vi "LSMcontroller_v57.vi"() -> ()   [LabVIEW 2015] (continued)
  out "graph1":dbl[](graph)=[-0.0018560309667373077, -0.0018495913478545844, -0.0010736164951231331, -0.001495411962387152, -0.0016886007197899743, -0.0017819752829382196, -0.002049219731125049, -0.0016853808861924334, -0.0013730590644991025, -0.0016853808995801955, -0.0015823469014139846, -0.0019494055502582341, -0.0022907056851545348, -0.0020041423733346162, -0.002042780100600794, -0.001814173402963206, -0.001997702724765986, -0.002136154668405652, -0.002451696299831383, -0.0024710151832550765, -0.0021297150413738565, -0.002165132985683158, -0.0019429659144952892, -0.0021908914903178813, -0.0024291576351970433, -0.002606247318908572, -0.0019204272195929661, -0.0018946687219431623, -0.002097516918438487, -0.0021844518574653192, -0.002290705653722398, -0.0020299008616711943, -0.001859250800916925, -0.0015630280249752104, -0.001852811174467206, -0.0017884149093879388, -0.001955845166812651, -0.0018302724667591975, -0.0012957835738779976, -0.0013923779356991872, -0.0015018515911651776, -0.0015404893353115768, -0.0016467431501951068, -0.0016789412929210813, -0.0015533685742411762, -0.0014116968284361064, -0.00147931290557608, -0.001682161101489328, -0.002023461216595024, -0.0021941113128559663, -0.0019429659086745233, -0.0014567741996143013, -0.0017916347202844918, -0.0021393744961824266, -0.0021941113081993535, -0.0022327490517636763, -0.0023132443812210112, -0.002129715041955933, -0.002149033914320171, -0.002216649982728995, -0.0024645755731035023, -0.002760798340314068, -0.0022295292594935747, -0.00198482348525431, -0.0021168357878923417, -0.002065318789682351, -0.0024259378161514177, -0.002239188695093617, -0.0022134301700862126, -0.001917207420920022, -0.0015469289664179087, -0.0017626564193051308, -0.0020459999179001896, -0.0021136160084279255, -0.0018689102173084394, -0.0013408609433099628, -0.0014406751602655276, -0.001495411946089007, -0.0016982601588824765, -0.001820613036979921, -0.0014213562669465319, -0.001437455345876515, -0.0012088486348511651, -0.0014503345714183525, -0.0016467431612545624, -0.0018012941704364494, -0.0016918205167166889, -0.0016596224083332345, -0.0016370837058639154, -0.0016950403252849356, -0.002084637672523968, -0.002326123615493998, -0.0023068047373089938, -0.0022585075575625524, -0.00199126310297288, -0.002107176355784759, -0.002165133003727533, -0.0026384454587241634, -0.0025676095741800965, -0.0025225321960169822, -0.0021264952316414564, -0.0020427801075857135, -0.0021200556465191768, -0.002245628290693276, -0.002390519853797741, -0.0022746066143736242, -0.0020910772954812274, -0.0017851950967451558, -0.0017465573363006114, -0.0018817894713720306, -0.0021619131858460604, -0.0017916347179561852, -0.001736897912924178, -0.0016048855806002392, -0.0013344213337404653, -0.0013794987014262006, -0.001804513976094313, -0.0018334922881331295, -0.0016821610782062635, -0.0012861241400241852, -0.0011605514463735745, -0.0016467431490309536, -0.0018334922892972827, -0.0017948545346735045, -0.0018528111593332142, -0.0015662478364538402, -0.0017948545276885851, -0.0018495913362130522, -0.00211683580360841, -0.0022907056659460068, -0.002065318794338964, -0.002100736728752963, -0.001965504598338157, -0.001923647031071596, -0.002380860450793989, -0.0025160925590898844, -0.0024516962975030766, -0.0021973311249166728, -0.0021425942954374478, -0.0021039565571118147, -0.002480674621765502, -0.0024581359419971706, -0.002406618939130567, -0.0020653187792049723, -0.0020331206818809734, -0.0019011083693476394, -0.0024066189402947202, -0.002100736736319959, -0.001959064974216744, -0.0016757214703829958, -0.0015243902738438918, -0.001749777131481096, -0.001827052648877725, -0.0015662478102603926, -0.0017046997835859657, -0.0015501487703295424, -0.0013891581393545493, -0.0013762788905296475, -0.0014213562599616125, -0.00181739320687484, -0.001666062013246119, -0.0017240186640992761, -0.0012829043267993257, -0.0016274242772487924, -0.0016821611020714044, -0.0021329348516883327, -0.0020009225263493136, -0.002216649993788451, -0.0018399319046875462, -0.0016950403217924758, -0.002116835783235729, -0.0023357830644818024, -0.002493553873500787, -0.002644885074696504, -0.0022230896214023234, -0.0021039565443061294, -0.00202668106299825, -0.002371201001224108, -0.002718940763734281, -0.0023583217366831377, -0.002239188690437004, -0.001988043275196105, -0.001933306478895247, -0.0023969594959635286, -0.002149033925961703, -0.0019333064742386341, -0.0017851950996555389, -0.0015662478434387594, -0.001572687451262027, -0.0017207988345762715, -0.001968724424368702, -0.001749777148361318, -0.0017111394059611484, -0.0011991891922662034, -0.0012957835855195298, -0.0015694676392013207, -0.0018431517033604904, -0.00160810538160149, -0.001669281840440817, -0.0014857525273691862, -0.001495411968207918, -0.0017143592133652419, -0.0020266810234170407, -0.0022295292478520423, -0.0019751640438335017, -0.0016821610962506383, -0.00206209899391979, -0.0020910772978095338, -0.0025579501484753564, -0.0023454424826195464, -0.0021651330019813032, -0.0020942971110343932, -0.0021264952316414564, -0.002206990561098792, -0.0025386312487535177, -0.0024323774583172053, -0.002242408492020331, -0.0021361546911066397, -0.0019429659011075274, -0.0021071763639338315, -0.0024806746386457235, -0.0022552877361886204, -0.0019333064934471621, -0.0015565884031821043, -0.0018656904040835797, -0.0017368979088496416, -0.0020620989764574913, -0.002004142368095927, -0.0018141734122764318, -0.0014471147704171016, -0.0011025947914458812, -0.0015501487709116192, -0.0018624705949332565, -0.0017948545253602787, -0.00177231585199479, -0.0013537401973735541, -0.0013698392553487793, -0.0016628422040957957, -0.0017401177121791989, -0.00198482348350808, -0.0020395603036740795, -0.0018399319052696229, -0.0015018515754491092, -0.0017916347266873345, -0.0021812320401659235, -0.00237764063233044, -0.002216649978654459, -0.002123275414924137, -0.001949405528139323, -0.0019977027032291516, -0.002387300063855946, -0.0025515104917576536, -0.002274606619030237, -0.002081417862791568, -0.002078198051312938, -0.001981603662716225, -0.002487114255782217, -0.002786556836217642, -0.0020588791550835593, -0.0017690960131585597, -0.001769096020143479, -0.0019300866511184722, -0.0021329348592553287, -0.0022681669978192077, -0.0018946687231073155, -0.0015147308318410068, -0.0013601798203308135, -0.0015630280249752104, -0.002039560312987305, -0.0021973311225883664, -0.00174977716000285, -0.0012957835773704574, -0.0012378269532928243, -0.0014342355192638935, -0.0020653187891002743, -0.0018399319058516994, -0.0015372695308178664, -0.001476093094679527, -0.00159200633817818, -0.0017690960387699306, -0.0017562167765572667, -0.0020331206731498243, -0.002190891476930119, -0.001936526307836175, -0.0016467431496130303, -0.0016338639007881283, -0.0022102103638462723, -0.0023776406107936052, -0.0023905198776628823, -0.002152253762469627, -0.001859250787529163, -0.002155473546590656, -0.00242593782953918, -0.0023357830609893426, -0.002393739692051895, -0.0021522537450073286, -0.00203634048870299, -0.0020041423657676206, -0.0021232754172524435, -0.0023390028806170447, -0.0022746066277613865, -0.001868910220800899, -0.0016692818503361195, -0.0017207988328300416, -0.001881789463222958, -0.0019429659412708133, -0.0020266810309840367, -0.0017272384563693777, -0.001334421323845163, -0.0012700250651687384, -0.001740117723820731, -0.0018656904302770273, -0.001794854526524432, -0.001469653451931663, -0.0015437091555213557, -0.0015791270794579758, -0.0017272384988609702, -0.0017529969615861774, -0.002013801789144054, -0.0020266810426255687, -0.0016821610735496507, -0.0016692818270530553, -0.0017723158199805767, -0.0023100245353998615, -0.002416278381133452, -0.002290705683408305, -0.0018689102382631973, -0.0017594366031698882, -0.0021876716788392513, -0.002458135940833017, -0.002361541569116525, -0.0023293434327933938, -0.0019526253320509568, -0.0018431517231510951, -0.0021168357849819584, -0.0024903340463060886, -0.00241305856325198, -0.002332563240779564, -0.001785195113043301, -0.001843151740031317, -0.0017980743205407634, -0.0019590649631572887, -0.00209751692134887, -0.0019880433013895527, -0.0015565884084207937, -0.0013633996300632134, -0.0015501487522851676, -0.0017143592156935482, -0.00209107730537653, -0.0016789412766229361, -0.0013666194613324478, -0.0013633996393764391, -0.0012668052542721853, -0.001556588388630189, -0.0019075479550519957, -0.0018238328368170187, -0.001756216786452569, -0.0014986317686270921, -0.0014277958963066339, -0.0017916347336722539, -0.0019397461105836555, -0.002210210368502885, -0.002132934860419482, -0.0018817894748644904, -0.0018656904192175716, -0.0019880432955687866, -0.002033120676060207, -0.0023551019409205763, -0.002467795368283987, -0.002052439529215917, -0.0018173932161880658, -0.0022166499897139148, -0.0023840802599443124, -0.0024581359291914852, -0.0024549161351751538, -0.0023712010233430192, -0.0020009225455578416, -0.0018334922770736738, -0.001942965938942507, -0.001939746110001579, -0.002329343447345309, -0.0020073621690971776, -0.0017916347255231813, -0.0015082911960780621, -0.00143423551809974, -0.0017240186623530462, -0.0019751640473259615, -0.0019107677799183875, -0.001572687461739406, -0.0012925637559965252, -0.0010736165021080523, -0.0015726874460233375, -0.0018270526523701846, -0.0018689102242933587, -0.001685380867565982, -0.0015501487615983934, -0.001347300586057827, -0.0016370837099384517, -0.0019977027317509056, -0.002097516935900785, -0.0020717584155499937, -0.0016757214447716252, -0.0018206130363978446, -0.0020814178476575764, -0.002345442486112006, -0.0026642039592843503, -0.002264947179937735, -0.0019043281738413498, -0.002161913178279065, -0.002149033920140937, -0.0024194981885375453, -0.0025579501315951348, -0.002306804757681675, -0.002007362169679254, -0.001933306460850872, -0.0021844518580473957, -0.002184451878420077, -0.002271386809879914, -0.00211039618588984, -0.00177231585199479, -0.0015759072575019673, -0.0017143592203501612, -0.0017111393983941525, -0.0019590649823658167, -0.001791634718538262, -0.0016435233206721022, -0.0011637712555238977, -0.001453554396284744, -0.0017336780938785523, -0.0016982601548079402, -0.0018656904180534184, -0.001563028022646904, -0.0011573316162684932, -0.0015726874658139422, -0.0014567742095096038, -0.0018721300427569077, -0.002107176362769678, -0.0019461857079295442, -0.0019397461030166597, -0.0018045139574678615, -0.0019204272172646598, -0.0019912631140323357, -0.002187671684077941, -0.0024291576375253497, -0.0023035849432926623, -0.0020653187989955767, -0.0020717584114754574, -0.002123275409685448, -0.0023390028876019643, -0.002622346395510249, -0.0023261236131656917, -0.002252067932859063, -0.001865690387203358, -0.0020041423477232456, -0.0021329348761355504, -0.0022778264153748753, -0.0021103961765766145, -0.001959064967231825, -0.001717579016694799, -0.0014986317593138664, -0.001627424283651635, -0.0018914489058079198, -0.0018367120838956906, -0.0014406751457136124, -0.0015501487586880103, -0.0013022232073126362, -0.001421356256469153, -0.0016982601478230208, -0.0015501487703295424, -0.0018045139615423978, -0.001582346884533763, -0.0013440807693405076, -0.0015179506508866325, -0.0018302724696695805, -0.002000922540901229, -0.0018431517150020228, -0.001823832843801938, -0.0017980743595398963, -0.0018817894667154179, -0.0019268668530276045, -0.0022424084757221865, -0.0026481048861751334, -0.002406618953682482, -0.002087857477017678, -0.0018431517371209339, -0.0024066189589211718, -0.0023647613829234615, -0.002284266062779352, -0.002499993511009961, -0.0021908914734376592, -0.001904328142409213, -0.0021071763546206056, -0.0021490339195588603, -0.002522532190196216, -0.002113615990965627, -0.0016499629808822648, -0.0016338638897286728, -0.0017368979076854885, -0.00202346122416202, -0.001852811149437912]
  in  "graph1list":u16(ring) items=["PMT"]
  out "Cmembrane":dbl
  in  "fitpoints":dbl=10.0
  out "Racces (MOhm)":dbl
  out "Rmembrane (MOhm)":dbl
  in  "set as Rp?":bool
  out "Ifit":dbl[](graph)
  in  "readpatch":bool
  in  "Voltage Clamp":bool=TRUE
  in  "OCgain":sgl(ring)=5.0 caption="Output Current gain (mV/pA)" items=["2K"=2000, "1K"=1000, "500"=500, "200"=200, "100"=100, "50"=50, "20"=20, "10"=10, "5"=5, "2"=2, "1"=1, "0.5"=0.5, "0.2"=0.2, "0.1"=0.1, "0.05"=0.05, "0.02"=0.02, "0.01"=0.01, "0.005"=0.005]
  in  "holdon":bool
  out "CC_ICgain":dbl(ring)=10.0 caption="Current Clamp \ninput current gain (pA/mV)" items=["0.1"=10.0, "10"=0.1]
  out "Patch readout":dbl[][](graph)=[[-19.129690948880636, -18.936502231865173, -19.129690948880636, -19.065294709927485, -19.065294709927485, -19.097492829410562, -19.065294709927485, -19.000898470922337, -19.065294709927485, -19.065294709927485, -19.097492829410562, -19.129690948880636, -19.065294709927485, -19.22628530721287, -19.065294709927485, -19.033096590431416, -19.000898470922337, -19.129690948880636, -19.065294709927485, -19.000898470922337, -19.097492829410562, -19.097492829410562, -19.129690948880636, -19.097492829410562, -19.065294709927485, -19.19408718778179, -18.96870035140026, -19.033096590431416, -19.097492829410562, -19.033096590431416, -19.065294709927485, -19.065294709927485, -19.129690948880636, -19.097492829410562, -19.129690948880636, -19.16188906833771, -19.065294709927485, -19.065294709927485, -19.16188906833771, -19.16188906833771, -19.065294709927485, -19.129690948880636, -19.097492829410562, -19.033096590431416, -19.065294709927485, -19.129690948880636, -19.065294709927485, -19.033096590431416, -19.033096590431416, -19.129690948880636, -19.19408718778179, -19.065294709927485, -9.148273285922594, -9.212669532972436, -9.180471409454158, -9.083877038819596, -9.148273285922594, -9.148273285922594, -9.083877038819596, -9.148273285922594, -9.180471409454158, -9.180471409454158, -9.180471409454158, -9.212669532972436, -9.212669532972436, -9.180471409454158, -9.212669532972436, -9.11607516237774, -9.244867656477426, -9.11607516237774, -9.212669532972436, -9.244867656477426, -9.244867656477426, -9.11607516237774, -9.148273285922594, -9.212669532972436, -9.148273285922594, -9.212669532972436, -9.212669532972436, -9.180471409454158, -9.180471409454158, -9.277065779969131, -9.309263903447553, -9.244867656477426, -9.180471409454158, -9.180471409454158, -9.148273285922594, -9.244867656477426, -9.212669532972436, -9.244867656477426, -9.083877038819596, -9.212669532972436, -9.277065779969131, -9.244867656477426, -9.180471409454158, -9.11607516237774, -9.180471409454158, -9.212669532972436, -9.212669532972436, -9.212669532972436, -9.11607516237774, -9.180471409454158, -19.065294709927485, -19.097492829410562, -19.097492829410562, -19.16188906833771, -19.16188906833771, -19.033096590431416, -19.065294709927485, -19.129690948880636, -19.129690948880636, -19.097492829410562, -19.033096590431416, -19.258483426630953, -19.129690948880636, -19.033096590431416, -19.097492829410562, -19.129690948880636, -19.097492829410562, -19.19408718778179, -19.16188906833771, -19.097492829410562, -19.033096590431416, -19.000898470922337, -19.065294709927485, -19.16188906833771, -19.129690948880636, -19.129690948880636, -19.065294709927485, -19.033096590431416, -19.097492829410562, -19.097492829410562, -19.097492829410562, -18.96870035140026, -19.097492829410562, -19.19408718778179, -19.097492829410562, -19.065294709927485, -19.097492829410562, -19.129690948880636, -19.16188906833771, -19.033096590431416, -19.065294709927485, -19.129690948880636, -19.129690948880636, -19.065294709927485, -19.065294709927485, -19.033096590431416, -19.16188906833771, -19.097492829410562, -19.19408718778179, -19.000898470922337, -9.148273285922594, -9.148273285922594, -9.148273285922594, -9.019480791663437, -9.180471409454158, -9.277065779969131, -9.148273285922594, -9.148273285922594, -9.180471409454158, -9.180471409454158, -9.11607516237774, -9.180471409454158, -9.180471409454158, -9.11607516237774, -9.083877038819596, -9.341462026912685, -9.180471409454158, -9.11607516237774, -9.11607516237774, -9.212669532972436, -9.11607516237774, -9.11607516237774, -9.083877038819596, -9.11607516237774, -9.180471409454158, -9.11607516237774, -9.11607516237774, -9.244867656477426, -9.180471409454158, -9.180471409454158, -9.244867656477426, -9.180471409454158, -9.180471409454158, -9.180471409454158, -9.180471409454158, -9.180471409454158, -9.148273285922594, -9.11607516237774, -9.180471409454158, -9.212669532972436, -9.180471409454158, -9.148273285922594, -9.083877038819596, -9.11607516237774, -9.180471409454158, -9.148273285922594, -9.148273285922594, -9.148273285922594, -9.212669532972436, -9.11607516237774, -19.000898470922337, -19.065294709927485, -19.097492829410562, -19.129690948880636, -19.097492829410562, -18.936502231865173, -18.96870035140026, -19.097492829410562, -19.065294709927485, -19.097492829410562, -19.22628530721287, -19.065294709927485, -19.000898470922337, -19.000898470922337, -19.16188906833771, -19.065294709927485, -18.96870035140026, -19.097492829410562, -19.129690948880636, -19.065294709927485, -19.097492829410562, -19.129690948880636, -19.129690948880636, -19.16188906833771, -19.129690948880636, -19.129690948880636, -19.065294709927485, -19.000898470922337, -19.065294709927485, -19.065294709927485, -19.129690948880636, -19.033096590431416, -19.129690948880636, -19.065294709927485, -19.129690948880636, -19.097492829410562, -18.96870035140026, -19.097492829410562, -19.097492829410562, -19.065294709927485, -19.097492829410562, -19.129690948880636, -19.000898470922337, -19.033096590431416, -19.097492829410562, -19.097492829410562, -19.033096590431416, -18.96870035140026, -19.000898470922337, -19.129690948880636, -9.019480791663437, -9.083877038819596, -9.11607516237774, -9.083877038819596, -9.148273285922594, -9.309263903447553, -9.148273285922594, -9.11607516237774, -9.180471409454158, -9.180471409454158, -9.148273285922594, -9.148273285922594, -9.212669532972436, -9.019480791663437, -9.180471409454158, -9.148273285922594, -9.212669532972436, -9.051678915248162, -9.180471409454158, -9.212669532972436, -9.148273285922594, -9.212669532972436, -9.148273285922594, -9.11607516237774, -9.180471409454158, -9.212669532972436, -9.11607516237774, -9.083877038819596, -9.180471409454158, -9.11607516237774, -9.148273285922594, -9.083877038819596, -9.244867656477426, -9.212669532972436, -9.11607516237774, -9.11607516237774, -9.11607516237774, -9.148273285922594, -9.11607516237774, -9.11607516237774, -9.148273285922594, -9.180471409454158, -9.180471409454158, -9.051678915248162, -9.083877038819596, -9.083877038819596, -9.244867656477426, -9.083877038819596, -9.051678915248162, -9.148273285922594, -19.065294709927485, -19.065294709927485, -19.000898470922337, -19.000898470922337, -19.097492829410562, -19.065294709927485, -19.000898470922337, -19.097492829410562, -19.097492829410562, -19.033096590431416, -19.033096590431416, -19.033096590431416, -19.000898470922337, -19.065294709927485, -18.936502231865173, -19.065294709927485, -19.129690948880636, -19.065294709927485, -19.033096590431416, -19.000898470922337, -19.033096590431416, -19.065294709927485, -19.033096590431416, -19.065294709927485, -19.065294709927485, -19.129690948880636, -19.065294709927485, -19.033096590431416, -19.097492829410562, -19.033096590431416, -19.033096590431416, -19.097492829410562, -19.065294709927485, -19.129690948880636, -19.000898470922337, -19.033096590431416, -19.065294709927485, -19.097492829410562, -19.000898470922337, -19.033096590431416, -19.033096590431416, -19.000898470922337, -19.033096590431416, -19.033096590431416, -19.033096590431416, -19.033096590431416, -19.16188906833771, -19.000898470922337, -19.065294709927485, -19.065294709927485, -9.212669532972436, -9.083877038819596, -9.051678915248162, -9.148273285922594, -9.148273285922594, -9.212669532972436, -9.148273285922594, -9.148273285922594, -9.11607516237774, -9.11607516237774, -9.11607516237774, -9.11607516237774, -9.083877038819596, -9.180471409454158, -9.083877038819596, -9.11607516237774, -9.11607516237774, -9.244867656477426, -9.083877038819596, -9.019480791663437, -9.083877038819596, -9.212669532972436, -9.148273285922594, -9.083877038819596, -9.11607516237774, -9.11607516237774, -9.083877038819596, -9.083877038819596, -9.083877038819596, -8.987282668065419, -9.083877038819596, -9.148273285922594, -9.180471409454158, -9.083877038819596, -9.11607516237774, -9.212669532972436, -9.212669532972436, -9.083877038819596, -9.180471409454158, -9.148273285922594, -9.180471409454158, -9.180471409454158, -9.212669532972436, -9.180471409454158, -9.180471409454158, -9.11607516237774, -9.180471409454158, -9.244867656477426, -9.148273285922594, -9.148273285922594, -19.097492829410562, -19.16188906833771, -19.097492829410562, -19.033096590431416, -19.097492829410562, -19.033096590431416, -19.065294709927485, -19.097492829410562, -19.065294709927485, -19.000898470922337, -19.000898470922337, -19.000898470922337, -19.000898470922337, -19.065294709927485, -19.097492829410562, -19.065294709927485, -19.033096590431416, -19.129690948880636, -19.19408718778179, -19.097492829410562, -19.033096590431416, -19.16188906833771, -19.097492829410562, -19.16188906833771, -19.129690948880636, -19.065294709927485, -19.065294709927485, -19.000898470922337, -19.16188906833771, -19.129690948880636, -19.065294709927485, -19.097492829410562, -19.129690948880636, -19.19408718778179, -19.097492829410562, -19.129690948880636, -19.097492829410562, -19.097492829410562, -19.16188906833771, -19.033096590431416, -19.097492829410562, -19.129690948880636, -19.033096590431416, -19.097492829410562, -19.129690948880636, -19.22628530721287, -19.16188906833771, -19.065294709927485, -19.033096590431416, -19.097492829410562, -9.180471409454158, -9.180471409454158, -9.277065779969131, -9.244867656477426, -9.212669532972436, -9.11607516237774, -9.083877038819596, -9.11607516237774, -9.244867656477426, -9.019480791663437, -9.148273285922594, -9.083877038819596, -9.148273285922594, -9.051678915248162, -9.148273285922594, -9.019480791663437, -9.180471409454158, -9.148273285922594, -9.148273285922594, -9.212669532972436, -9.083877038819596, -8.987282668065419, -9.11607516237774, -9.212669532972436, -9.244867656477426, -9.083877038819596, -9.083877038819596, -9.083877038819596, -9.148273285922594, -9.148273285922594, -9.11607516237774, -9.212669532972436, -9.148273285922594, -9.148273285922594, -9.180471409454158, -9.019480791663437, -9.148273285922594, -9.180471409454158, -9.083877038819596, -9.083877038819596, -9.180471409454158, -9.212669532972436, -9.083877038819596, -9.11607516237774, -9.180471409454158, -9.180471409454158, -9.11607516237774, -9.180471409454158], [-35.779977141471754, -40.28771474745375, -34.49205210635021, -34.1700708472335, -34.81403336533239, -37.067902174441265, -37.71186469011919, -35.45799588289315, -36.423939658225486, -35.136014624180035, -37.067902174441265, -41.253658516736806, -35.779977141471754, -35.136014624180035, -40.609696004015795, -41.89762102892044, -34.49205210635021, -35.45799588289315, -35.779977141471754, -35.779977141471754, -36.74592091640061, -32.88214580942104, -38.677808462627745, -35.136014624180035, -35.45799588289315, -37.71186469011919, -34.49205210635021, -34.81403336533239, -36.101958399915866, -37.71186469011919, -39.64375223392652, -38.35582720525932, -37.067902174441265, -39.96573349075733, -35.136014624180035, -39.64375223392652, -40.28771474745375, -38.033845947756475, -32.23818328970733, -36.74592091640061, -35.45799588289315, -34.49205210635021, -34.49205210635021, -40.609696004015795, -37.38988343234745, -34.49205210635021, -34.49205210635021, -37.71186469011919, -39.64375223392652, -39.64375223392652, -33.84808958798223, -34.81403336533239, 678.0528204855508, 1131.0810610228193, 502.25090087551973, 199.266378015621, 75.94752772468436, 25.074483129972915, 3.1797561257887312, -5.5137382458773425, -15.817138854881982, -15.817138854881982, -17.105063921275384, -19.68091404758065, -19.68091404758065, -16.78308265487962, -19.68091404758065, -15.49515758794595, -13.88525125123923, -14.529213786327267, -18.071007719652435, -18.392988985508072, -17.105063921275384, -16.461101388348812, -13.56326998349251, -18.071007719652435, -17.74902645366178, -17.105063921275384, -20.9688391074937, -12.275344911154063, -18.071007719652435, -19.036951516814337, -18.071007719652435, -18.714970251228706, -15.49515758794595, -15.49515758794595, -19.036951516814337, -15.49515758794595, -21.612801636640594, -12.919307447593619, -11.953363642731512, -18.071007719652435, -15.173176320874825, -13.56326998349251, -15.817138854881982, -15.49515758794595, -17.74902645366178, -18.714970251228706, -13.88525125123923, -15.173176320874825, -18.714970251228706, -15.173176320874825, -733.5130643686014, -1187.5061495938146, -557.3894460524117, -254.08323998283743, -130.76444258972012, -71.84187725332792, -51.87903989910548, -42.863564796188484, -39.64375223392652, -38.677808462627745, -39.32177097696133, -41.89762102892044, -38.999789719861745, -33.20412706907601, -37.38988343234745, -37.38988343234745, -35.779977141471754, -38.35582720525932, -36.423939658225486, -33.84808958798223, -37.067902174441265, -33.52610832859641, -32.23818328970733, -37.38988343234745, -38.033845947756475, -34.81403336533239, -39.32177097696133, -40.28771474745375, -35.136014624180035, -37.067902174441265, -38.35582720525932, -34.1700708472335, -36.423939658225486, -35.779977141471754, -34.49205210635021, -37.71186469011919, -36.74592091640061, -33.84808958798223, -35.45799588289315, -34.81403336533239, -33.52610832859641, -36.101958399915866, -38.999789719861745, -44.15148981733241, -35.779977141471754, -34.81403336533239, -32.88214580942104, -41.89762102892044, -34.49205210635021, -33.20412706907601, 674.8330046967607, 1133.9788972951085, 500.9629748915052, 201.52024753339165, 76.59149033645211, 24.43052056204702, -0.6840191627033408, -12.597326179441428, -12.275344911154063, -10.987419836652661, -14.529213786327267, -22.578745429349105, -19.036951516814337, -12.919307447593619, -17.74902645366178, -15.173176320874825, -16.461101388348812, -20.324876577807075, -13.241288715610644, -14.8511950536686, -14.529213786327267, -13.88525125123923, -15.49515758794595, -19.036951516814337, -19.036951516814337, -12.597326179441428, -21.612801636640594, -24.83261427428173, -16.461101388348812, -12.597326179441428, -17.74902645366178, -15.49515758794595, -14.20723251885081, -17.105063921275384, -15.817138854881982, -16.139120121682932, -20.324876577807075, -17.74902645366178, -17.105063921275384, -16.139120121682932, -19.35893278226498, -17.105063921275384, -20.00289531276134, -18.392988985508072, -17.74902645366178, -13.56326998349251, -16.78308265487962, -21.29082037213461, -20.646857842717857, -12.597326179441428, -730.615235463241, -1184.6083220554708, -557.3894460524117, -256.01512699731944, -130.12048015097793, -78.92546457817109, -55.09885241038406, -42.21960228481076, -41.5756397728958, -38.033845947756475, -35.45799588289315, -36.74592091640061, -34.81403336533239, -39.32177097696133, -34.1700708472335, -35.45799588289315, -38.033845947756475, -34.81403336533239, -38.35582720525932, -37.067902174441265, -34.49205210635021, -35.45799588289315, -38.999789719861745, -39.32177097696133, -41.5756397728958, -37.067902174441265, -33.84808958798223, -37.71186469011919, -37.38988343234745, -35.136014624180035, -39.64375223392652, -34.81403336533239, -38.999789719861745, -36.101958399915866, -38.35582720525932, -38.35582720525932, -38.033845947756475, -41.5756397728958, -40.93167726044347, -33.84808958798223, -33.52610832859641, -31.916202029648574, -37.38988343234745, -37.38988343234745, -32.23818328970733, -38.35582720525932, -36.423939658225486, -38.677808462627745, -34.1700708472335, -34.49205210635021, 678.6967836451707, 1128.8271883760178, 499.35306741486363, 196.6905271466478, 77.55743425513697, 26.040426982883794, 1.5698497532110507, -12.275344911154063, -15.817138854881982, -11.631382374173768, -12.275344911154063, -18.071007719652435, -16.78308265487962, -20.00289531276134, -20.9688391074937, -16.461101388348812, -19.036951516814337, -16.461101388348812, -16.139120121682932, -19.35893278226498, -16.78308265487962, -19.68091404758065, -13.56326998349251, -15.173176320874825, -16.461101388348812, -21.612801636640594, -18.071007719652435, -13.88525125123923, -17.105063921275384, -17.4270451875361, -13.241288715610644, -13.88525125123923, -20.324876577807075, -19.036951516814337, -17.4270451875361, -16.461101388348812, -21.612801636640594, -16.461101388348812, -19.036951516814337, -18.392988985508072, -13.241288715610644, -16.78308265487962, -20.646857842717857, -16.139120121682932, -13.241288715610644, -10.987419836652661, -13.88525125123923, -23.222707957147, -16.139120121682932, -17.4270451875361, -732.2251404118074, -1186.540207081943, -556.4235028932625, -250.21946594002904, -128.51057405181638, -80.8573520192037, -56.38677741114458, -43.82950856224784, -38.677808462627745, -35.136014624180035, -34.1700708472335, -38.033845947756475, -33.84808958798223, -37.067902174441265, -35.45799588289315, -38.999789719861745, -37.067902174441265, -38.999789719861745, -38.677808462627745, -41.89762102892044, -37.067902174441265, -35.779977141471754, -35.45799588289315, -36.423939658225486, -34.49205210635021, -34.1700708472335, -43.82950856224784, -37.38988343234745, -32.88214580942104, -36.74592091640061, -37.71186469011919, -33.20412706907601, -36.423939658225486, -34.1700708472335, -36.423939658225486, -38.677808462627745, -35.779977141471754, -38.35582720525932, -37.38988343234745, -35.45799588289315, -35.136014624180035, -27.086483112608153, -38.033845947756475, -40.93167726044347, -34.49205210635021, -38.35582720525932, -39.32177097696133, -39.64375223392652, -39.32177097696133, -37.38988343234745, 679.340746805411, 1135.910788150883, 504.50477135332426, 202.80817297522802, 79.1673407890343, 21.854670295792648, -3.5818506162647887, -11.309401105480822, -6.157700787998381, -12.275344911154063, -20.646857842717857, -17.105063921275384, -13.241288715610644, -16.139120121682932, -17.105063921275384, -19.036951516814337, -18.714970251228706, -16.461101388348812, -21.93478290101167, -14.8511950536686, -13.56326998349251, -17.105063921275384, -12.275344911154063, -14.20723251885081, -19.036951516814337, -16.139120121682932, -17.105063921275384, -19.68091404758065, -12.275344911154063, -19.68091404758065, -22.256764165247834, -16.461101388348812, -15.173176320874825, -17.74902645366178, -18.392988985508072, -15.817138854881982, -16.461101388348812, -22.256764165247834, -16.139120121682932, -15.49515758794595, -11.953363642731512, -18.714970251228706, -21.612801636640594, -17.74902645366178, -11.631382374173768, -16.139120121682932, -15.817138854881982, -17.74902645366178, -15.49515758794595, -11.953363642731512, -735.1229693120254, -1187.1841687566255, -553.5256734093635, -255.04918349065514, -131.08642380889358, -77.63753961481774, -57.67470240976262, -42.21960228481076, -37.067902174441265, -36.101958399915866, -39.96573349075733, -38.999789719861745, -33.84808958798223, -36.74592091640061, -38.35582720525932, -38.35582720525932, -38.35582720525932, -38.999789719861745, -35.45799588289315, -36.101958399915866, -38.999789719861745, -40.609696004015795, -35.136014624180035, -38.033845947756475, -42.54158354056677, -31.272239509127207, -39.64375223392652, -35.45799588289315, -31.916202029648574, -34.1700708472335, -39.64375223392652, -38.033845947756475, -31.5942207694552, -37.38988343234745, -40.28771474745375, -35.779977141471754, -34.81403336533239, -35.136014624180035, -35.45799588289315, -35.136014624180035, -37.067902174441265, -38.35582720525932, -36.423939658225486, -35.45799588289315, -35.45799588289315, -37.71186469011919, -38.677808462627745, -38.677808462627745, -38.35582720525932, -31.916202029648574, 679.6627283857648, 1130.7590792156293, 502.8948638684274, 203.4521356969947, 73.69365858783573, 23.142595427830134, 0.9258872051291477, -4.22581316001062, -12.597326179441428, -15.173176320874825, -18.714970251228706, -20.646857842717857, -16.461101388348812, -17.74902645366178, -15.49515758794595, -15.49515758794595, -16.139120121682932, -16.461101388348812, -15.817138854881982, -16.139120121682932, -19.036951516814337, -11.631382374173768, -12.597326179441428, -15.173176320874825, -18.071007719652435, -19.35893278226498, -19.036951516814337, -15.49515758794595, -18.714970251228706, -15.817138854881982, -20.00289531276134, -17.74902645366178, -16.78308265487962, -16.139120121682932, -13.88525125123923, -16.139120121682932, -19.35893278226498, -21.612801636640594, -12.275344911154063, -20.324876577807075, -18.714970251228706, -17.74902645366178, -12.597326179441428, -15.49515758794595, -17.74902645366178, -21.29082037213461, -12.275344911154063, -13.88525125123923]]
  in  "Vholding (mV)":sgl caption="Vhold (mV)" step=0.1 format="%_6g"
  in  "sealtest":bool
  in  "Current Clamp":bool
  out "Rpipette (MOhm)":dbl
  out "Sampling rate \ncurrent wf":dbl
  out "remDO":bool
  out "addDO":bool
  in  "refwf":u32(ring)=3 caption="reference waveforms to:" items=["X", "Y", "2P pockels cell", "640 AO", "488 AO", "532 AO", "Voltage to Patch", "Voltage to Zpos", "2p Shutter", "488 shutter", "camera trigger", "640 shutter", "LT timestamp", "640 blanking", "488 blanking", "532 blanking", "2P ODfilt trigger ", "LCVR"]
  out "remAO":bool
  out "addAO":bool
  in  "Add AO wave":bool
  out "Analog Used Lines":tag[](array[tag])
  in  "Rem AO wave":bool
  in  "Add DO wave":bool
  in  "Build digital waveform tabs":enum32{"Simple", "Matlab"}(tab)
  in  "Digital time offset (s)":dbl
  in  "Digital padding value":dbl
  in  "Digital phase (s)":dbl
  in  "Digital DC (%)":dbl=50.0
  in  "Digital Freq (Hz)":dbl=50.0
  in  "Matlab padding value DO":dbl caption="Matlab padding value"
  in  "Load Matlab Waveform DO":bool
  in  "Matlab waveform path DO":path caption="Matlab waveform path"
  out "Digital Used Lines":tag[](array[tag])
  in  "Rem DO wave":bool
  out "Total Camera Frames":i32=-1
  out "Digital Lines Plot":digitalwaveform[](graph)
  out "Analog Lines Plot":waveform(dbl)[](graph)
  in  "Build analog waveform tabs":enum32{"Square", "Triangle", "Matlab"}(tab)
  in  "padding value":dbl
  in  "Start amplitude (V)":dbl=1.0
  in  "Period (ms)":dbl=1000.0
  in  "DC (%)":dbl=100.0
  in  "Step size (V)":dbl=1.0
  in  "Baseline (V)":dbl
  in  "Cycles":dbl=5.0
  in  "Repeats":dbl=1.0
  in  "phase shift (ms)":dbl=1.0
  in  "Pulses":dbl=1.0
  in  "Tri padding value":dbl
  in  "Tri Phase (s)":dbl
  in  "Tri Repeats":dbl
  in  "Frequency":dbl
  in  "Offset (V)":dbl
  in  "Amplitude (V)":dbl
  in  "Matlab padding value":dbl
  in  "Load Matlab Waveform":bool
  in  "Matlab waveform path":path
  out "Digital Used Names":string[](array[string])
  out "Analog Used Names":string[](array[string])
  in  "AO channels":u32(ring)=3 items=["X", "Y", "2P pockels cell", "640 AO", "488 AO", "532 AO", "Voltage to Patch", "Voltage to Zpos"]
  in  "DO channels":u16(ring) items=["2p Shutter", "488 shutter", "camera trigger", "640 shutter", "LT timestamp", "640 blanking", "488 blanking", "532 blanking", "2P ODfilt trigger ", "LCVR"]
  in  "Loaded settings":u16(ring) items=["citrinecomp"]
  in  "Setting location":path=path "C:/Users/Labmember/Desktop/Temp Data/2015-04-07 (Neurons DIV7 retigabine)/150957_Dish1_Cell07_1p5OD_p2"
  in  "Nickname":string="Pulse1"
  in  "Add settings":bool
  in  "Rem setting":bool
  in  "Update settings":bool
  in  "Bin size":T7(ring)
  out "Histogram 2":u32[](graph)
  out "Integral count":u32
  out "Lifetime (ns)":dbl
  in  "Input Method":u16(ring) items=["Unbinned", "Binned"]
  out "Ch1Rate":i32(slide) scale=0.01..100000000.0 scale format="%.0e"
  out "SyncRate":i32(slide) scale=0.01..100000000.0 scale format="%.0e"
  out "Histogram":u32[](graph)
  in  "Ch1 Level":i32=300 min=0 max=800 step=10
  in  "Ch1 ZeroX":i32=10 min=0 max=20 step=1
  in  "Ch0 ZeroX":i32=10 min=0 max=20 step=1
  in  "Ch0 Level":i32=70 min=0 max=800 step=10
  out "Save tab":enum32{"withsave", "withoutsave"}(tab)
  in  "save\ndata":bool=TRUE
  in  "filename prefix":string
  out "data dir":path=path "C:/Users/Labmember/Desktop/Data/temp" caption="save folder for data of current measurement"
  in  "AI channels":i32[](listbox)=[4]
  in  "avpp":i32=1 caption="# averages\n per point" min=1 step=1
  in  "# of frames":i32=1 min=1 step=1
  out "Current Average":sgl=1.0
  # "Waveform generation needs to be fixed in all \nprep channel subvis."
  # "Sampling"
  # "Dataset"
  # "Hardware controls"
  # "Stage Joystick"
  # "Manual Coordinates"
  # "ROI Coordinates"
  # "Manual Coordinates"
  # "ROI Coordinates"
  # "Z-Scan"
  # "Patch controls"
  # "Patch mode"
  # "resting potential:\nHEKcells: -20 to -40 mV\n(down to -70 mV offset to get gigaseal)\nNeurons: -70 mV"
  # "Patch mode"
  # "determine R,C"
  # "Set gains (OC gain must equal  'Gain' on HEKA!!)"
  # "input Voltage for voltage clamp and monitored output Voltage are always amplified by a factor 10 compared to voltage over pipette --> factor implemented outomatically in VC input, and in in display here, raw output data are saved"
  # "OCG has three modes \nwith different noise, bandwidth and feedback resistor characteristics\nLow gain: 0.005-0.2 -->large currents, loose patch, large cells --> CC input gain=10 pA/mV\nMedium gain 0.5-20 --> normal whole cell recordings --> CC input gain = 0.1 pA/mV\nHigh gain 50-2K --> single channel --> current clamp not possible"
  # "DON'T FORGET TO CLOSE PICOHARP\nDON'T FORGET TO TURN ON 1040"
  # "should be O(1)"
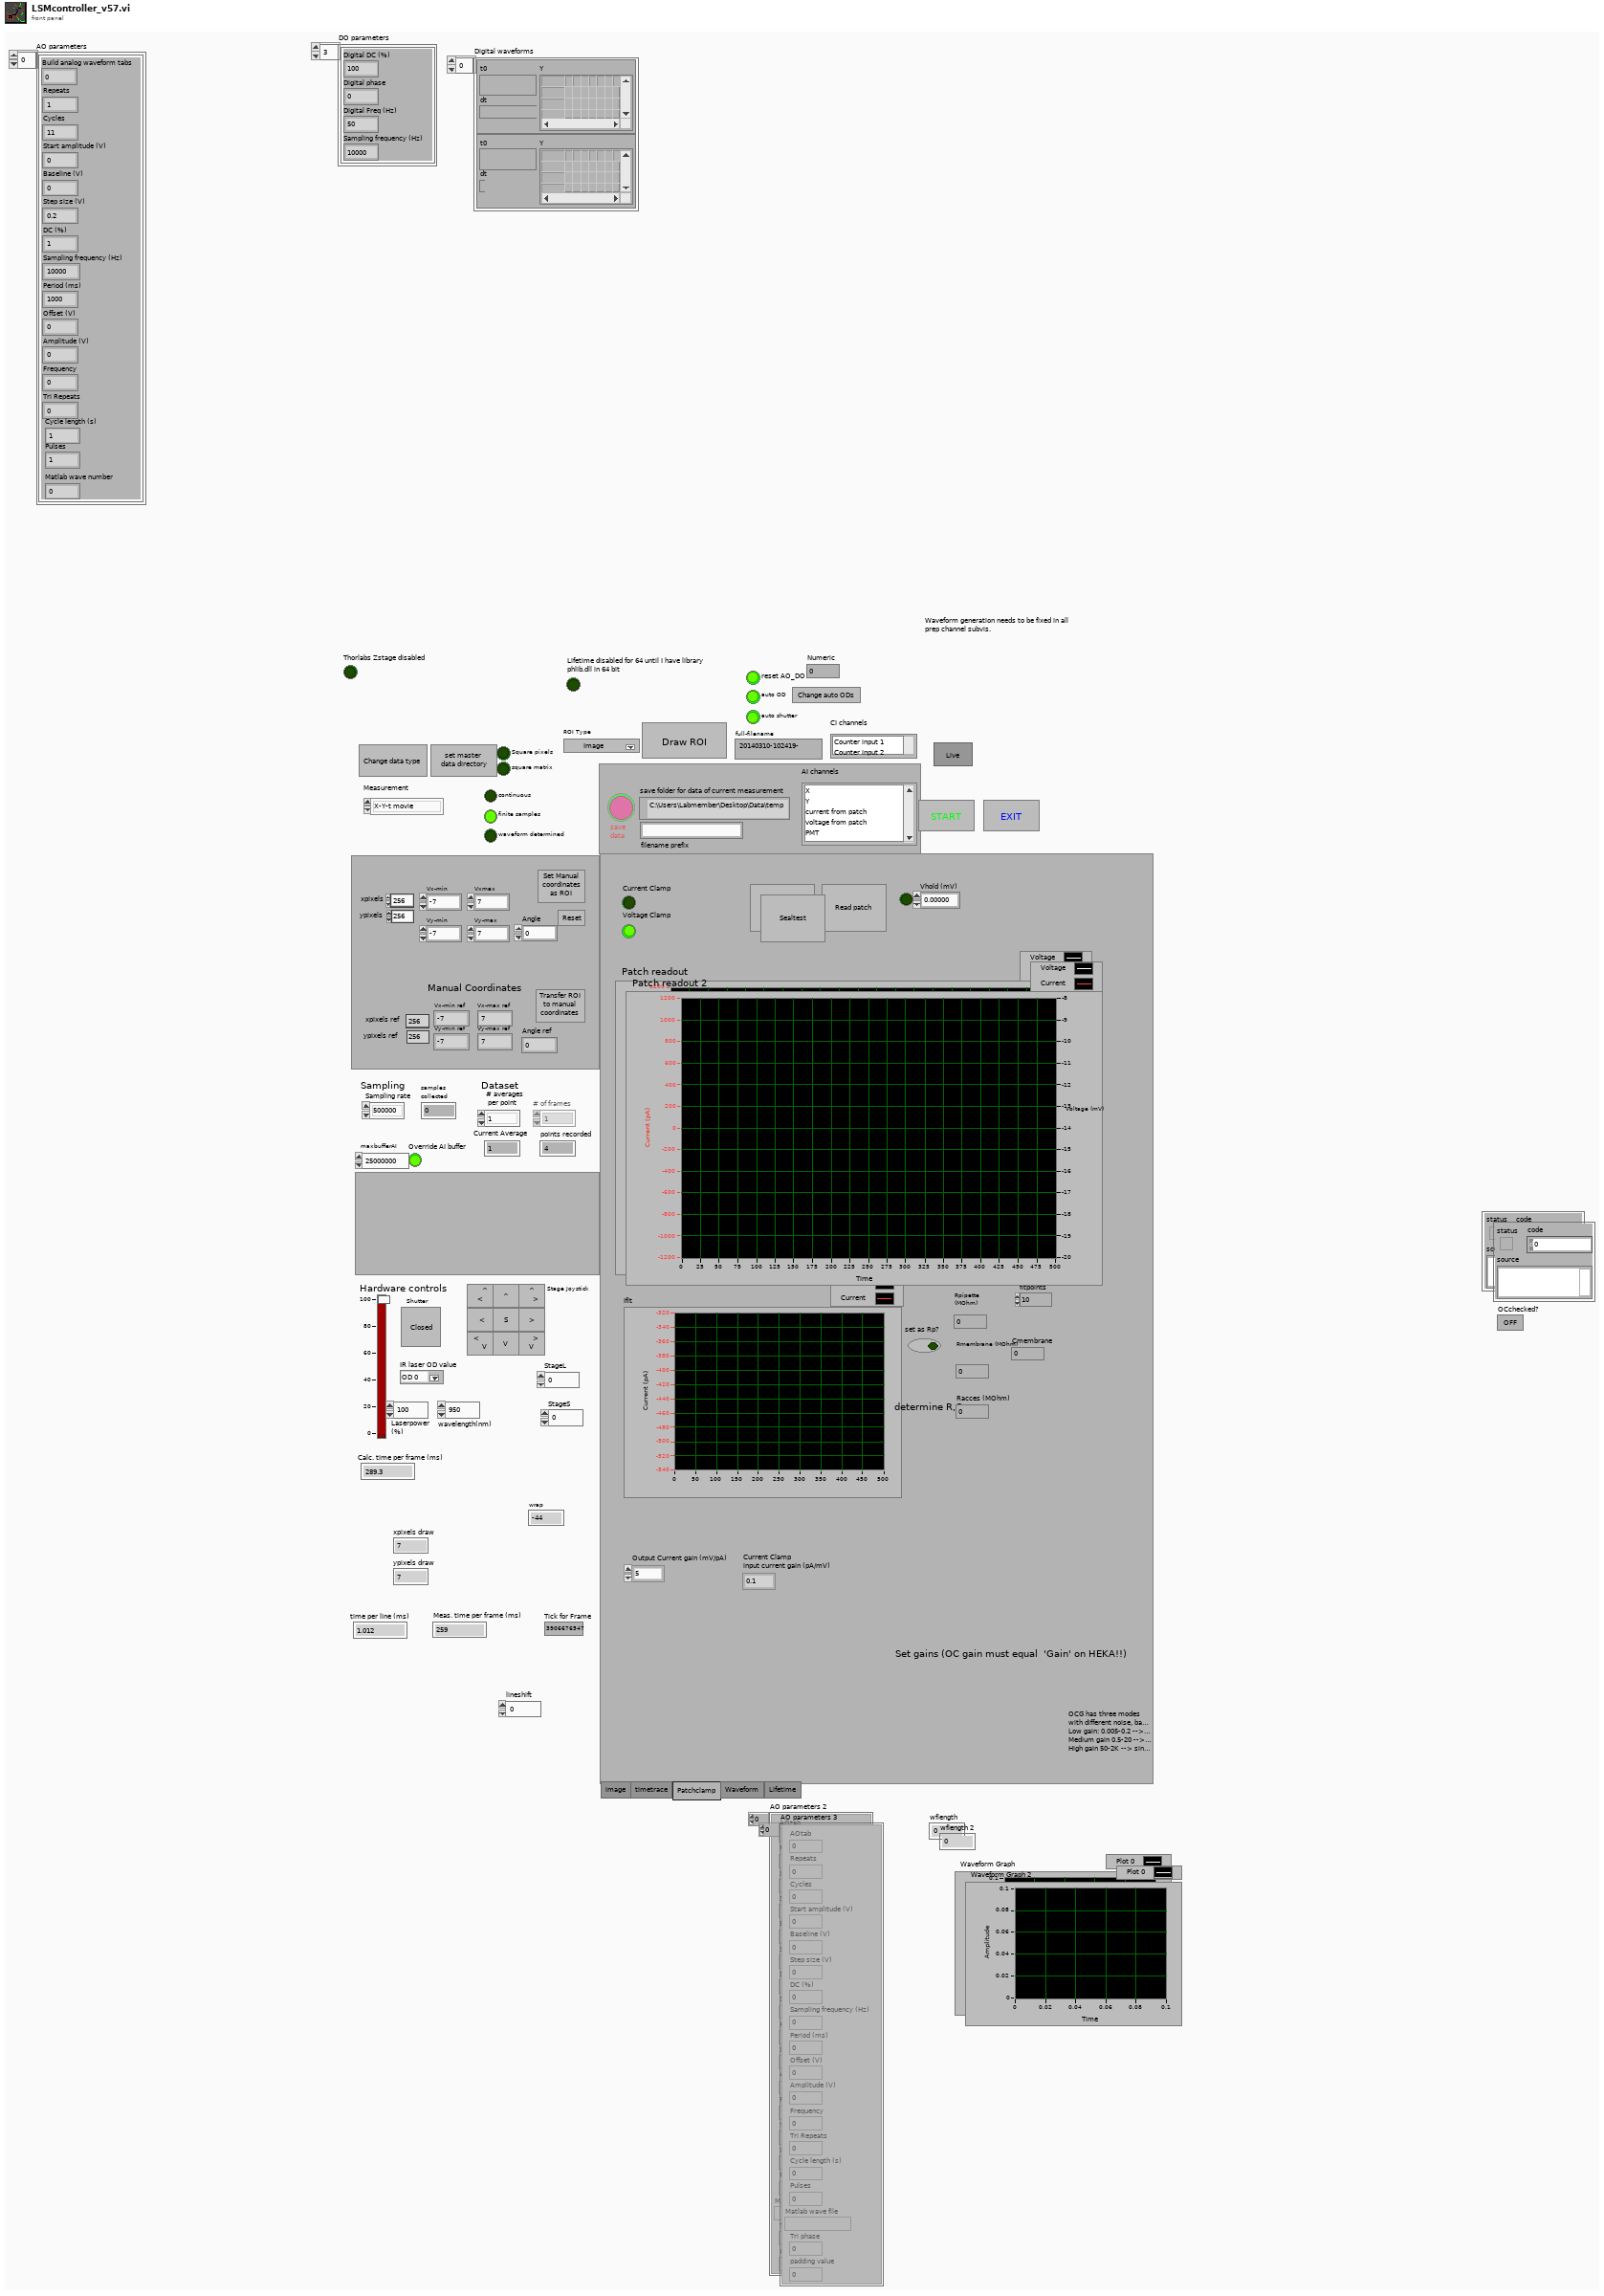
[diagram p1: front panel]
types:
  T1 = cluster{"AOtab":dbl, "Repeats":dbl, "Cycles":dbl, "Start amplitude (V)":dbl, "Baseline (V)":dbl, "Step size (V)":dbl, "DC (%)":dbl, "Sampling frequency (Hz)":dbl, "Period (ms)":dbl, "Offset (V)":dbl, "Amplitude (V)":dbl, "Frequency":dbl, "Tri Repeats":dbl, "Cycle length (s)":dbl, "Pulses":dbl, "Matlab wave file":path, "Tri phase":dbl, "padding value":dbl}[]
  T2 = cluster{"Digital DC (%)":dbl, "Digital phase":dbl, "Digital Freq (Hz)":dbl, "Sampling frequency (Hz)":dbl}[]
  T3 = cluster{"Build analog waveform tabs":dbl, "Repeats":dbl, "Cycles":dbl, "Start amplitude (V)":dbl, "Baseline (V)":dbl, "Step size (V)":dbl, "DC (%)":dbl, "Sampling frequency (Hz)":dbl, "Period (ms)":dbl, "Offset (V)":dbl, "Amplitude (V)":dbl, "Frequency":dbl, "Tri Repeats":dbl, "Cycle length (s)":dbl, "Pulses":dbl, "Matlab wave number":dbl}[]
  T4 = enum16{"Point", "Resonant Ellipse", "Line", "freeform contour"}
  T5 = enum16{"X-Y-t movie", "X-Y-Z stack", "X-Y-Z-t movie", "linescan", "Timetrace", "Lifetime (point)", "Lifetime (scan)", "Lifetime (contour)"}
  T6 = enum32{"image", "timetrace", "Patchclamp", "Waveform", "Lifetime"}
  T7 = enum16{"1", "2", "4", "8", "16", "32", "64", "128"}
  T8 = enum8{"Enabled", "Disabled", "Disabled and Grayed Out"}
  T9 = enum16{"open", "replace", "create", "open or create", "replace or create", "replace or create with confirmation"}
  T10 = enum16{"sealtest hekcells", "sealtest neurons", "Manual", "from file"}
  T11 = typedef "LVRectTypeDef.ctl" = cluster{"Left":i16, "Top":i16, "Right":i16, "Bottom":i16}
  T12 = cluster{"Xpixels":i32, "Vxminref":dbl, "Vxmaxref":dbl, "P":dbl, "Ypixels":i32, "Vyminref":dbl, "Vymaxref":dbl, "srate":sgl, "sAOxy":i32, "timeout":dbl, "type":string, "date":string, "time":string, "Colormap":u16, "Drawing Mode":u16, "Scanning Mode":u16, "square pixels":bool, "square matrix":bool, "Xpixels Img":i32, "Vx-min Img":dbl, "VX-max Img":dbl, "Ypixels Img":i32, "Vy-min Img":dbl, "Vy-max Img ":dbl, "Angle Img":dbl, "autoshutter":bool, "finite":bool, "cont":bool, "wavdet":bool, "measpoints":i32, "avpp":i32, "bufferAO":i32, "bufferAI":i32, "starttick":u32, "waveform":path, "Vx-ref":dbl, "Vy-ref":dbl, "refreshrate":dbl, "refreshbuffer":i32, "tt_cycles":i32, "motorref":refnum<k7>, "mirrorswitch":refnum<k7>, "sample mode":i32, "maxbufferAI":i32, "srateAODO":sgl, "bin":sgl, "Pel":sgl, "Angle draw":dbl, "srate Img":sgl, "ROIimg_plotbounds":T11, "auto OD":bool, "ODfilt":u16, "aAI":i32[], "aCI":i32[], "aAO":u32[], "aDO":u32[], "refwfsize":dbl, "Lifetime":bool, "Vz-Img":dbl, "Vz-ref":dbl, "Vz-reset":dbl, "AIoverride":bool}
  T13 = cluster{"StageS":i32, "StageL":i32, "currmeas data dir":path, "image OD":u16, "contour OD":u16, "point OD":u16, "AOlines":tag[], "AIlines":tag[], "CI lines":tag[], "DO lines":tag[], "AO names":string[], "CI names":string[], "AI names":string[], "DO names":string[], "CIextensions":string[], "AIextensions":string[], "Voltage to Ygalvo":i32, "Voltage to Xgalvo":i32, "Voltage to patch":i32, "640 shutter":i32, "2P shutter":i32, "LT timestamp":u32, "Vp":i32, "Ip":i32, "camera trigger":i32, "master data dir":path, "voltage to Zpos":i32, "Vto2P":i32, "640 AO":i32, "488 AO":i32, "532 AO":i32, "640TTL":u32, "488TTL":u32, "532TTL":u32, "Device 1 sampleclock out":tag, "Device 1 Starttrigger out":tag, "Device 2 sampleclock in":tag, "Device 2 StartTrigger in ":tag, "2PODTTL":u32, "488 shutter":u32, "LCVR":u32}
  T14 = enum16{"Left Button", "Center Button", "Right Button", "Window Close"}
  T15 = cluster{"VC":bool, "CC":bool, "CC_icg (pA/mv)":sgl, "VC_icg (mV/mV)":sgl, "OCG (mV/pA)":sgl, "OVG (mV/mV)":dbl, "Vhold (mV)":sgl, "holdon":bool}
  T16 = cluster{"AO parameters":cluster{"AOtab":dbl, "Repeats":dbl, "Cycles":dbl, "Start amplitude (V)":dbl, "Baseline (V)":dbl, "Step size (V)":dbl, "DC (%)":dbl, "Sampling frequency (Hz)":dbl, "Period (ms)":dbl, "Offset (V)":dbl, "Amplitude (V)":dbl, "Frequency":dbl, "Tri Repeats":dbl, "phase shift (ms)":dbl, "Pulses":dbl, "Matlab wave file":path, "Tri phase":dbl, "padding value":dbl}[], "DO parameters":cluster{"Digital DC (%)":dbl, "Digital phase":dbl, "Digital Freq (Hz)":dbl, "Sampling frequency (Hz)":dbl, "Digital time offset (s) ":dbl, "padding value":dbl, "matlab wave file":path, "DOtab":dbl}[]}
  T17 = cluster{"AOtab":dbl, "Repeats":dbl, "Cycles":dbl, "Start amplitude (V)":dbl, "Baseline (V)":dbl, "Step size (V)":dbl, "DC (%)":dbl, "Sampling frequency (Hz)":dbl, "Period (ms)":dbl, "Offset (V)":dbl, "Amplitude (V)":dbl, "Frequency":dbl, "Tri Repeats":dbl, "phase shift (ms)":dbl, "Pulses":dbl, "Matlab wave file":path, "Tri phase":dbl, "padding value":dbl}[]
  T18 = cluster{"AOtab":dbl, "Repeats":dbl, "Cycles":dbl, "Start amplitude (V)":dbl, "Baseline (V)":dbl, "Step size (V)":dbl, "DC (%)":dbl, "Sampling frequency (Hz)":dbl, "Period (ms)":dbl, "Offset (V)":dbl, "Amplitude (V)":dbl, "Frequency":dbl, "Tri Repeats":dbl, "phase shift (ms)":dbl, "Pulses":dbl, "Matlab wave file":path, "Tri phase":dbl, "padding value":dbl}
  T19 = cluster{"Digital DC (%)":dbl, "Digital phase":dbl, "Digital Freq (Hz)":dbl, "Sampling frequency (Hz)":dbl, "Digital time offset (s) ":dbl, "padding value":dbl, "matlab wave file":path, "DOtab":dbl}[]
  T20 = cluster{"Digital DC (%)":dbl, "Digital phase":dbl, "Digital Freq (Hz)":dbl, "Sampling frequency (Hz)":dbl, "Digital time offset (s) ":dbl, "padding value":dbl, "matlab wave file":path, "DOtab":dbl}
  T21 = cluster{"initialized":bool, "devidx":i32, "Ch0 Level":i32, "Ch0 ZeroX":i32, "Ch1 Level":i32, "Ch1 ZeroX":i32, "sync rate":i32, "resolution":i32, "acq time":i32, "acq rate":i32, "# bins":u32, "Bin size":enum16{"1", "2", "4", "8", "16", "32", "64", "128"}, "min photons":u32, "truncate":u32}
  T22 = cluster{"upleft":bool, "up":bool, "upright":bool, "right":bool, "downright":bool, "down":bool, "downleft":bool, "left":bool, "Bigsmall":bool, "E_stage":errorcluster}
  T23 = typedef "DialogType.ctl" = u16
  T24 = cluster{"AO parameters":cluster{"Build analog waveform tabs":dbl, "Repeats":dbl, "Cycles":dbl, "Start amplitude (V)":dbl, "Baseline (V)":dbl, "Step size (V)":dbl, "DC (%)":dbl, "Sampling frequency (Hz)":dbl, "Period (ms)":dbl, "Offset (V)":dbl, "Amplitude (V)":dbl, "Frequency":dbl, "Tri Repeats":dbl, "Cycle length (s)":dbl, "Pulses":dbl, "Matlab wave number":dbl}[], "DO parameters":cluster{"Digital DC (%)":dbl, "Digital phase":dbl, "Digital Freq (Hz)":dbl, "Sampling frequency (Hz)":dbl}[]}
  T25 = cluster{"AO parameters":cluster{"AOtab":dbl, "Repeats":dbl, "Cycles":dbl, "Start amplitude (V)":dbl, "Baseline (V)":dbl, "Step size (V)":dbl, "DC (%)":dbl, "Sampling frequency (Hz)":dbl, "Period (ms)":dbl, "Offset (V)":dbl, "Amplitude (V)":dbl, "Frequency":dbl, "Tri Repeats":dbl, "Cycle length (s)":dbl, "Pulses":dbl, "Matlab wave file":path, "Tri phase":dbl, "padding value":dbl}[]}
  T26 = cluster{"AOtab":dbl, "Repeats":dbl, "Cycles":dbl, "Start amplitude (V)":dbl, "Baseline (V)":dbl, "Step size (V)":dbl, "DC (%)":dbl, "Sampling frequency (Hz)":dbl, "Period (ms)":dbl, "Offset (V)":dbl, "Amplitude (V)":dbl, "Frequency":dbl, "Tri Repeats":dbl, "Cycle length (s)":dbl, "Pulses":dbl, "Matlab wave file":path, "Tri phase":dbl, "padding value":dbl}
  T27 = cluster{"AO":refnum<k21>[], "E_AO":errorcluster[]}
  T28 = cluster{" AI":refnum<k21>, "E_AI":errorcluster, "header":dbl[]}
  T29 = cluster{"settings names":string[], "settings locations":path[]}
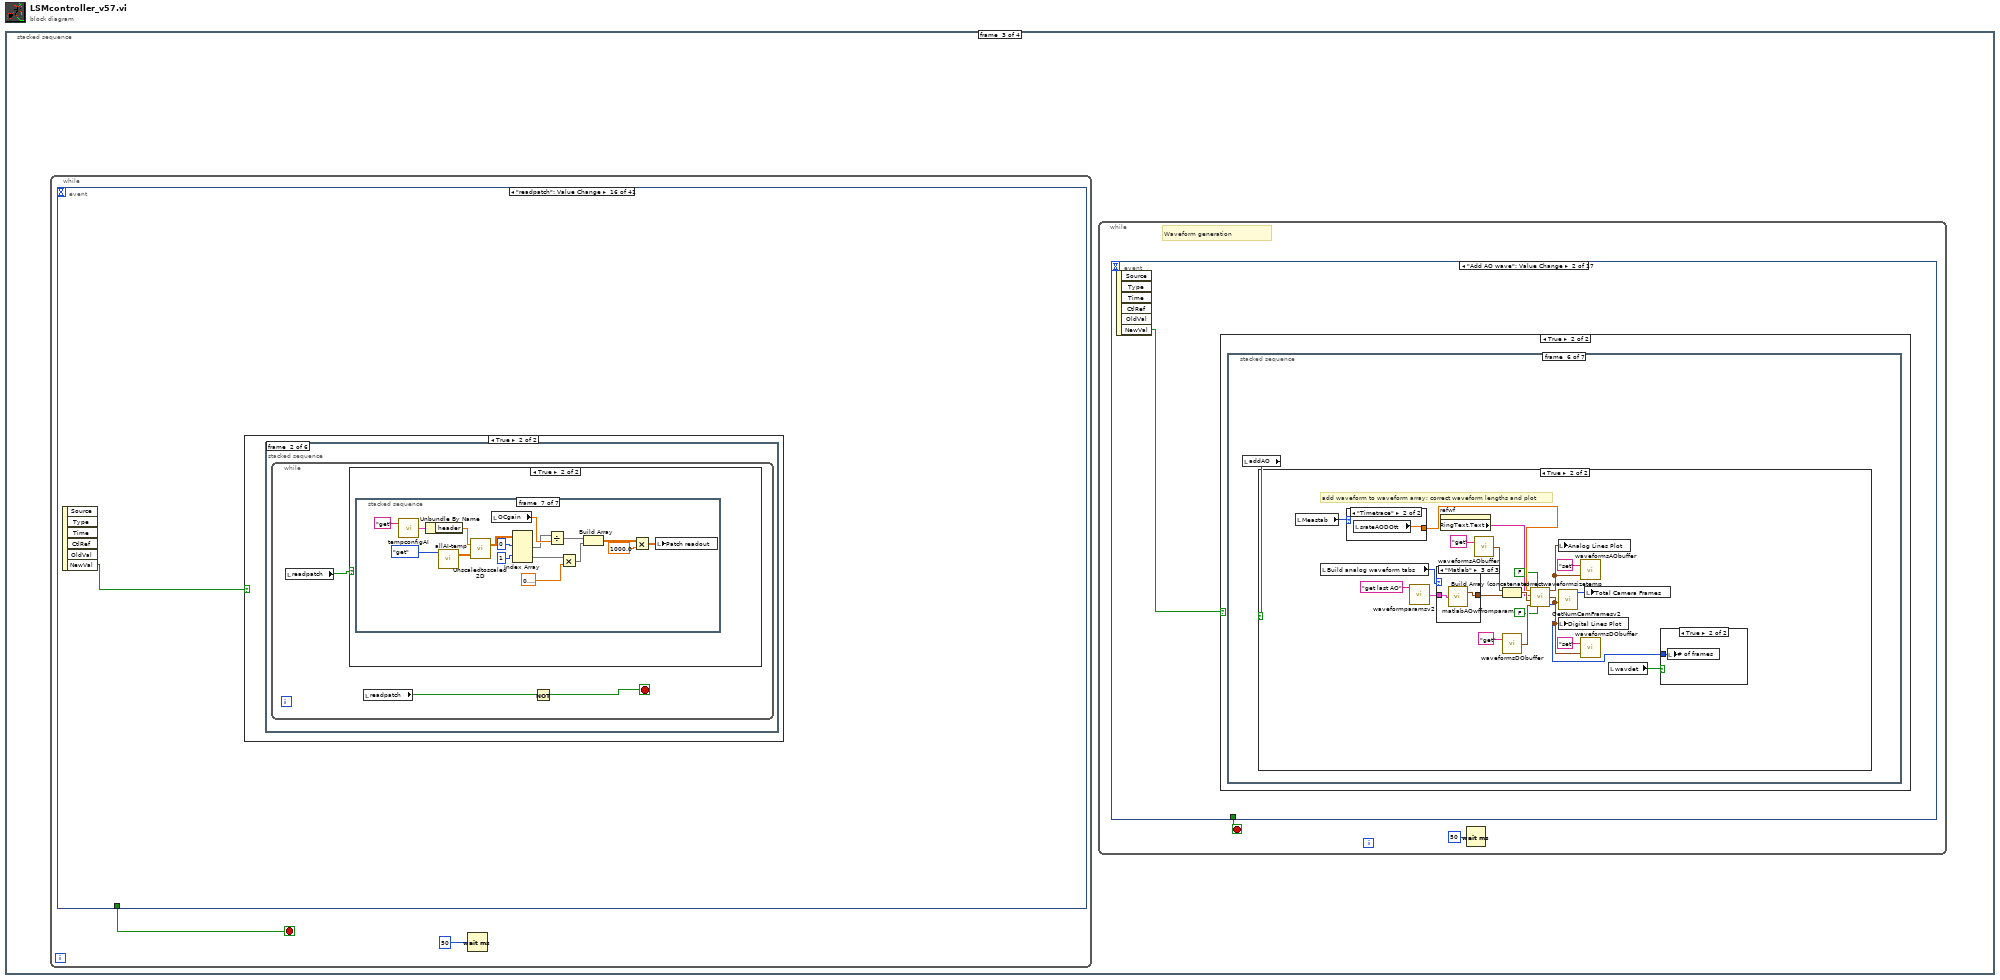
[diagram p0: block diagram]
diagram:
  n1 = stacked-sequence {
    frame #0 {
      "OCchecked?" <- FALSE ("Boolean")
    }
    frame #1 {
      w15 = u16 0 items=["Rectangle", "Circle", "Freeform Boundary", "Freeform Interior"] ("ROI Type")
      w24 = FALSE ("Value (Signaling)")
